vi "Add Label to Namer.vi"(10 "Label":string, 11 "Options in":refnum<class "Options.lvclass">) -> (3 "Options out":refnum<class "Options.lvclass">)   [LabVIEW 2020, in "Approval Tests.lvlib" / "Options.lvclass"]
uses:
  Options.lvclass
  Options.lvclass/Options.ctl
  Naming Data/Naming Data.lvclass/Naming Data.ctl
  Naming Data/Write Test Label.vi
  Naming Data/Naming Data.lvclass
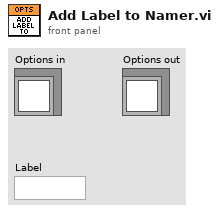
[diagram p1: front panel]
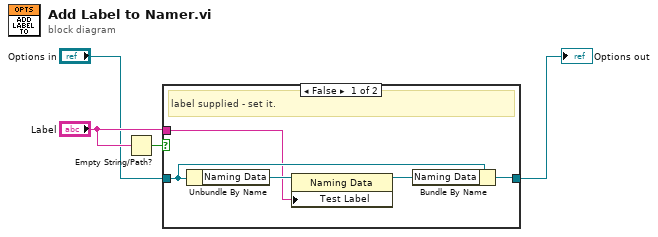
[diagram p0: block diagram]
diagram:
  n1 = Empty String/Path?(string/path="Label") -> (empty?=w4:bool)
  n2 = case shown="False" w4 {
    tunnel: "Label" -> [w5 _]
    tunnel: "Options in" -> [w6 w10]
    tunnel: [w7 w10] -> w1
    frame False {
      # "label supplied - set it."
      n3 = Unbundle By Name(w6) -> ("Naming Data"=w9:refnum<class "Naming Data.lvclass">)
      n4 = property on="Property Node" class="Naming Data"(reference=w9, "Test Label"=w5) -> (reference out=w8:refnum<class "Naming Data.lvclass">)  [unwired: 1 in, 1 out]
      n5 = Bundle By Name(cluster=w6, "Naming Data"=w8) -> (w7:refnum<class "Options.lvclass">)
    }
    frame True {
      # "label not supplied - don't change it."
    }
  }
  "Options out" <- w1
